vi "Log.vi"(8 "error in (no error)":errorcluster, 10 "Log Text":string, 11 "File Sink in":refnum<class "File Sink.lvclass">) -> (0 "error out":errorcluster, 3 "File Sink out":refnum<class "File Sink.lvclass">)   [LabVIEW 2020, in "LV Log.lvlib" / "File Sink.lvclass"]
uses:
  File Sink.lvclass
  File Sink.lvclass/File Sink.ctl
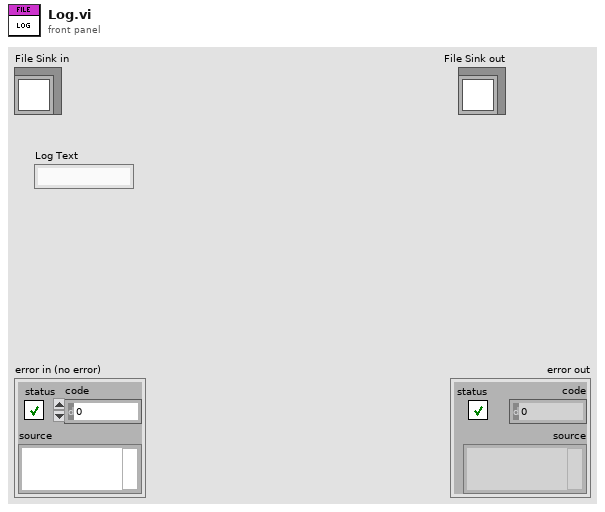
[diagram p1: front panel]
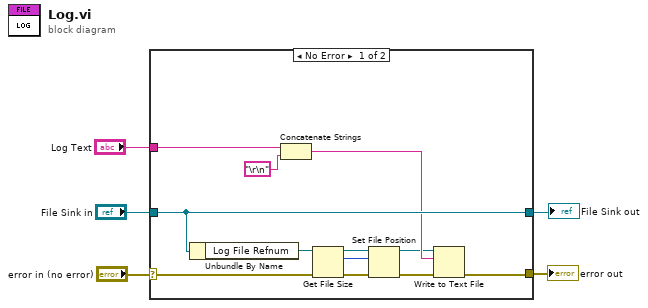
[diagram p0: block diagram]
diagram:
  n1 = case shown="No Error" "error in (no error)" {
    selector: "error in (no error)" -> [w7 w18]
    tunnel: [w16 w18] -> w4
    tunnel: [w17 w19] -> w3
    tunnel: "File Sink in" -> [w17 w19]
    tunnel: "Log Text" -> [w15 _]
    frame No Error {
      n2 = Unbundle By Name(w17) -> ("Log File Refnum"=w12:refnum<file>)
      n3 = Concatenate Strings(w15, "\r\n") -> (w14:string)
      n4 = Get File Size(file=w12, error in=w7) -> (refnum out=w11:refnum<file>, size (in bytes)=w6:i64, 0:w10:errorcluster)
      n5 = Set File Position(offset (in bytes) (0)=w6, refnum=w11, error in=w10) -> (refnum out=w9:refnum<file>, error out=w8:errorcluster)  [unwired: 1 in]
      n6 = Write to Text File(file (use dialog)=w9, text=w14, error in=w8) -> (error out=w16:errorcluster)  [unwired: 1 in, 2 out]
    }
    frame Error {
    }
  }
  "error out" <- w4
  "File Sink out" <- w3
